vi "VariablesTCValueChange.vi"(8 "error in (no error)":errorcluster, 10 "ValueChangeIn":T1, 11 "VMUI in":refnum<class "VMUI.lvclass">) -> (0 "error out":errorcluster, 3 "VMUI out":refnum<class "VMUI.lvclass">)   [LabVIEW 2013, in "VMUI.lvclass"]
uses:
  VMUI.lvclass
  API/VariableManagerAPI.lvlib
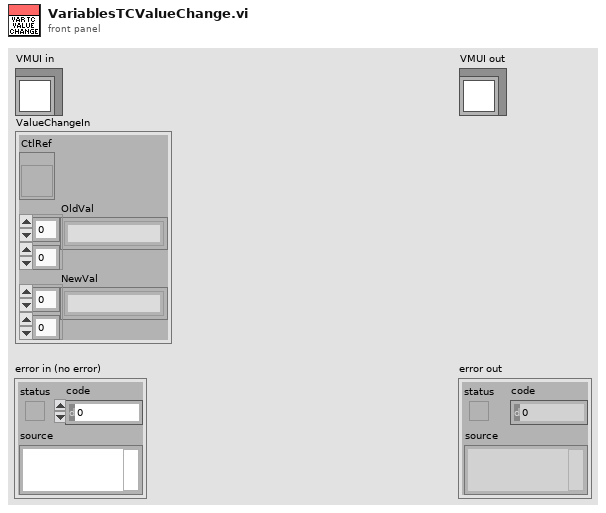
[diagram p1: front panel]
types:
  T1 = cluster{"CtlRef":refnum<vi>, "OldVal":string[][], "NewVal":string[][]}
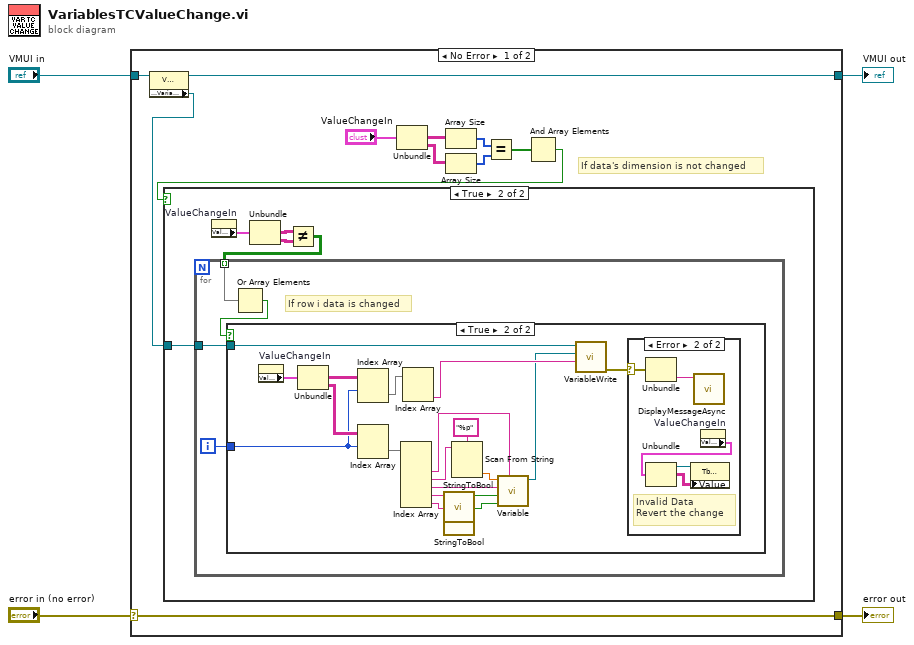
[diagram p0: block diagram]
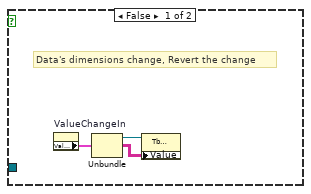
[diagram p2: hidden frame]
diagram:
  n1 = case shown="No Error" "error in (no error)" {
    selector: "error in (no error)" -> [w15 w53]
    tunnel: [w15 w53] -> w3
    tunnel: [w6 w52] -> w1
    tunnel: "VMUI in" -> [w7 w52]
    frame No Error {
      # "If data's dimension is not changed"
      n2 = property class="VMUI.lvclass"(reference=w7) -> (reference out=w6:refnum<class "VMUI.lvclass">, "Accessors:VariableManagerRef"=w5:refnum<vi>)  [unwired: 1 in, 1 out]
      n3 = Unbundle("ValueChangeIn") -> ("OldVal"=w13:string[][], "NewVal"=w14:string[][])  [unwired: 1 out]
      n4 = Array Size(array=w13) -> (size(s)=w8:i32[])
      n5 = Array Size(array=w14) -> (size(s)=w9:i32[])
      n6 = Equal?(x=w8, y=w9) -> (x = y?=w10:bool[])
      n7 = And Array Elements(Boolean array=w10) -> (logical AND=w11:bool)
      n8 = case shown="True" w11 {
        tunnel: w5 -> [_ w19]
        frame False {
          # "Data's dimensions change, Revert the change"
          n9 = property on="ValueChangeIn" class="Clust (strict)"() -> ("Value"=w18:T1)  [unwired: 2 in, 2 out]
          n10 = Unbundle(w18) -> ("CtlRef"=w17:refnum<vi>, "OldVal"=w16:string[][])  [unwired: 1 out]
          n11 = property class="Tbl (strict)"(reference=w17, "Value"=w16) -> ()  [unwired: 1 in, 2 out]
        }
        frame True {
          n12 = property on="ValueChangeIn" class="Clust (strict)"() -> ("Value"=w23:T1)  [unwired: 2 in, 2 out]
          n13 = Unbundle(w23) -> ("OldVal"=w22:string[][], "NewVal"=w21:string[][])  [unwired: 1 out]
          n14 = Not Equal?(x=w22, y=w21) -> (x != y?=w20:bool[][])
          n15 = for {
            tunnel: w20 -> [w27] mode=indexing
            tunnel: w19 -> [w24]
            i -> [w25]
            # "If row i data is changed"
            n16 = Or Array Elements(Boolean array=w27) -> (logical OR=w26:bool)
            n17 = case shown="True" w26 {
              tunnel: w25 -> [_ w40]
              tunnel: w24 -> [_ w29]
              frame False {
                # "No change"
              }
              frame True {
                n18 = property on="ValueChangeIn" class="Clust (strict)"() -> ("Value"=w46:T1)  [unwired: 2 in, 2 out]
                n19 = Unbundle(w46) -> ("OldVal"=w41:string[][], "NewVal"=w45:string[][])  [unwired: 1 out]
                n20 = Index Array(array=w41, index (row)=w40) -> (element=w39:string[])  [unwired: 1 in]
                n21 = Index Array(array=w45, index (row)=w40) -> (element=w44:string[])  [unwired: 1 in]
                n22 = Index Array(array=w44) -> (element #2=w36:string, element #3=w37:string, element #4=w34:string, element #5=w42:string, element #6=w43:string)  [unwired: 6 in, 1 out]
                n23 = Index Array(array=w39) -> (element #2=w31:string)  [unwired: 2 in, 1 out]
                n24 = call "StringToBool.vi"("StringIn"=w42) -> ("Boolean"=w33:bool)  [unwired: 10 in]
                n25 = call "StringToBool.vi"("StringIn"=w43) -> ("Boolean"=w32:bool)  [unwired: 10 in]
                n26 = Scan From String(format string="%p", input string=w37) -> (output 1=w35:dbl)  [unwired: 3 in, 3 out]
                n27 = call "Variable.vi"("VariableName"=w36, "InformIgor"=w32, "Sequence"=w33, "SequenceFunction"=w34, "DefaultValue"=w35) -> ("Variable"=w28:refnum<class "Variable.lvclass">)  [unwired: 6 in]
                n28 = call "VariableWrite.vi"("OriginalName"=w31, "Variable"=w28, "VariableManagerRef in"=w29) -> ("error out"=w30:errorcluster)  [unwired: 7 in, 1 out]
                n29 = case shown="Error" w30 {
                  selector: w30 -> [_ w48]
                  frame No Error {
                  }
                  frame Error {
                    # "Invalid Data\nRevert the change"
                    n30 = Unbundle(w48) -> ("source"=w47:string)  [unwired: 2 out]
                    n31 = call "DisplayMessageAsync.vi"("Message"=w47) -> ()  [unwired: 11 in]
                    n32 = property on="ValueChangeIn" class="Clust (strict)"() -> ("Value"=w51:T1)  [unwired: 2 in, 2 out]
                    n33 = Unbundle(w51) -> ("CtlRef"=w50:refnum<vi>, "OldVal"=w49:string[][])  [unwired: 1 out]
                    n34 = property class="Tbl (strict)"(reference=w50, "Value"=w49) -> ()  [unwired: 1 in, 2 out]
                  }
                }
              }
            }
          }
        }
      }
    }
    frame Error {
    }
  }
  "error out" <- w3
  "VMUI out" <- w1
